vi "Save File General Data.vi"(0 "Data File Path In":path, 1 "New File (Path Change)":bool, 2 "File Size":dbl=6.0 format="%#_13g", 5 "File Name Output Array":string[][](array[string]), 7 "Calibration Output Array":string[][](array[string]), 9 "Save Data":string[][](array[string]), 11 "Error In":errorcluster) -> (4 "Data File Path Out":path, 6 "New File":bool, 15 "Error Out":errorcluster)   [LabVIEW 2020]
uses:
  Save File.lvlib
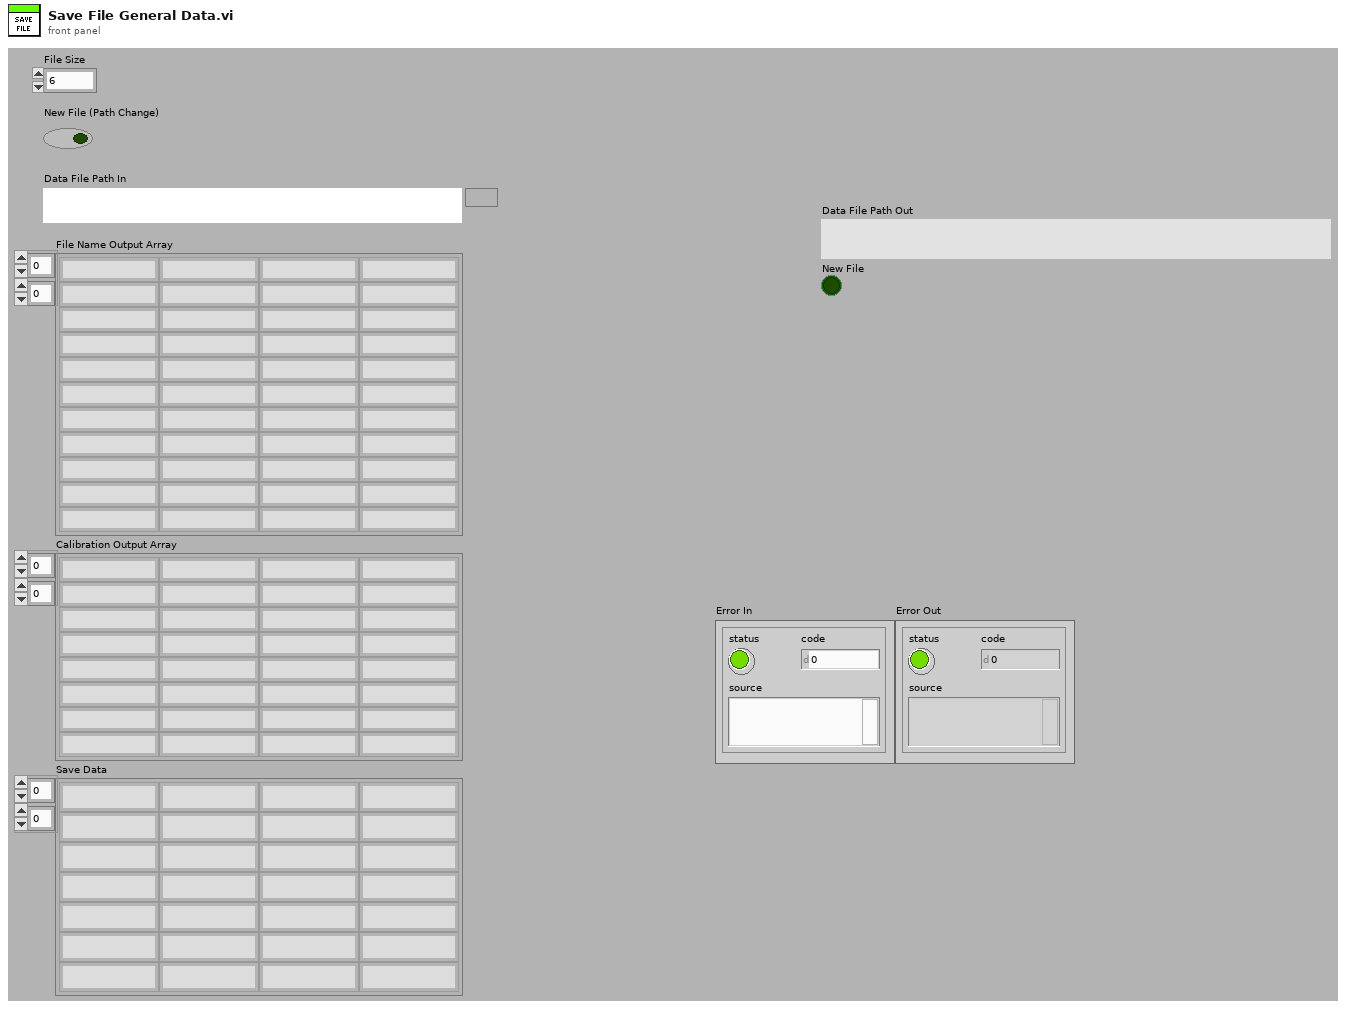
[diagram p1: front panel]
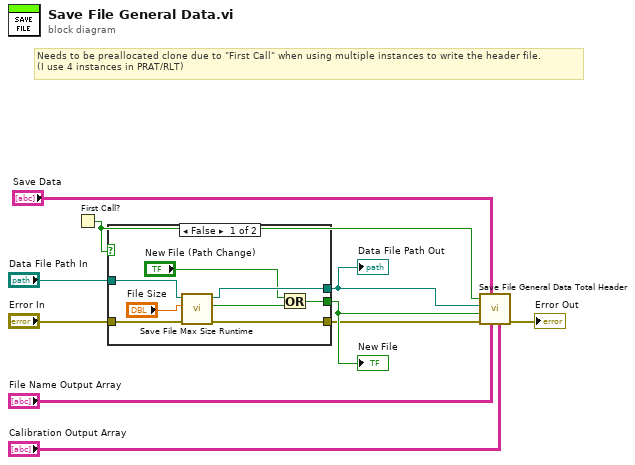
[diagram p0: block diagram]
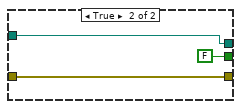
[diagram p2: hidden frame]
diagram:
  # "Needs to be preallocated clone due to \"First Call\" when using multiple instances to write the header file.\n(I use 4 instances in PRAT/RLT)"
  n1 = First Call?() -> (First Call?: T/F=w9:bool)
  n2 = case shown="False" w9 {
    tunnel: [w17 w21] -> w7
    tunnel: "Data File Path In" -> [w16 w21]
    tunnel: [w11 FALSE ("New File")] -> w8
    tunnel: "Error In" -> [w15 w19]
    tunnel: [w14 w19] -> w2
    frame False {
      n3 = call "Save File Max Size Runtime.vi"("Error In"=w15, "File Size"="File Size", "Old path"=w16) -> ("Error Out"=w14:errorcluster, "New File"=w13:bool, "New Path"=w17:path)  [unwired: 6 in]
      n4 = Or(x="New File (Path Change)", y=w13) -> (x .or. y?=w11:bool)
    }
    frame True {
    }
  }
  "New File" <- w8
  "Data File Path Out" <- w7
  n5 = call "Save File General Data Total Header.vi"("Calibration Output Array"="Calibration Output Array", "File Name Output Array"="File Name Output Array", "Save Data"="Save Data", "Error In"=w2, "New File"=w8, "Data File Path In"=w7, "First Call?: T/F"=w9) -> ("Error Out"=→"Error Out":errorcluster)  [unwired: 1 in, 3 out]
